vi "Example3_Week2.vi"() -> ()   [LabVIEW 2015]
panel:
  out "Waveform Chart":dbl(graph)
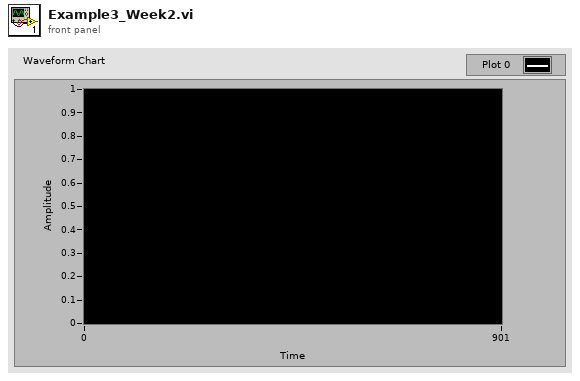
[diagram p1: front panel]
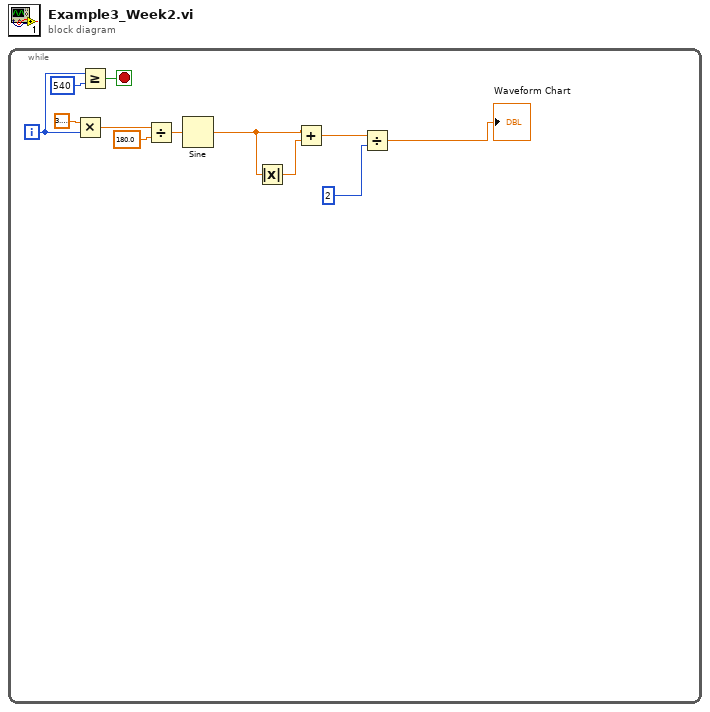
[diagram p0: block diagram]
diagram:
  n1 = while {
    i -> [w9]
    stop <- w7 stop-if-true
    n2 = Multiply(x=3.141592653589793, y=w9) -> (x*y=w10:dbl)
    n3 = Greater Or Equal?(x=w9, y=540) -> (x >= y?=w7:bool)
    n4 = Divide(x=w10, y=180.0) -> (x/y=w6:dbl)
    n5 = Sine(x=w6) -> (sin(x)=w5:dbl)
    n6 = Absolute Value(x=w5) -> (abs(x)=w4:dbl)
    n7 = Add(x=w5, y=w4) -> (x+y=w3:dbl)
    n8 = Divide(x=w3, y=2) -> (x/y=→"Waveform Chart":dbl)
  }
